vi "FuncImg-Export full data.vi"() -> (0 "error out":errorcluster, 11 "Exported file path":path)   [LabVIEW 2020]
uses:
  <userlib>/_MGI/File/MGI Windows Folder Enum.ctl
  Experiment header interface/Typedefs/Header parameters cluster-Zstack.ctl
  Typedefs/Frame Size.ctl
  Global variables/gl_Functional Imaging-Global variables.vi
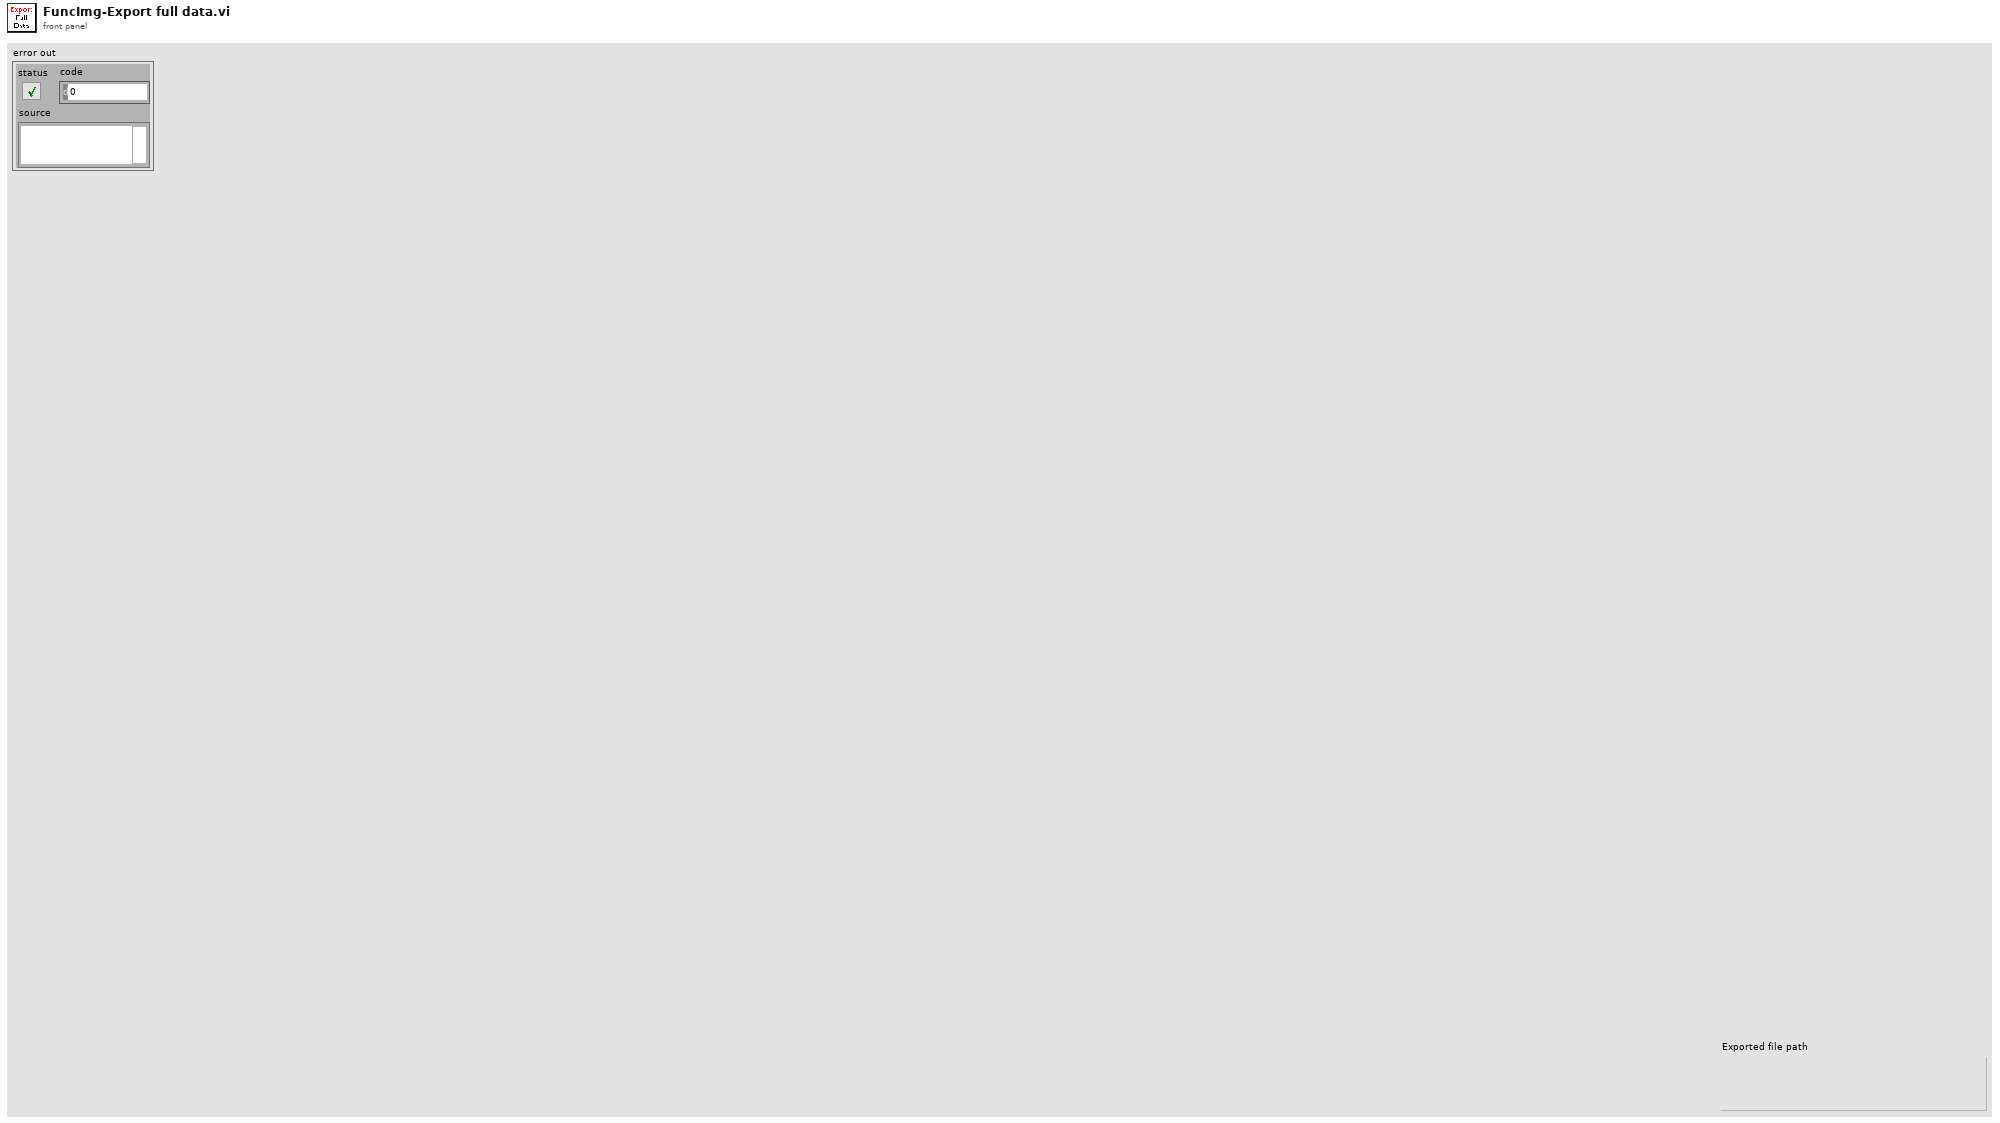
[diagram p1: front panel]
types:
  T1 = typedef "MGI Windows Folder Enum.ctl" = enum32{"Desktop", "Err<Internet>", "Programs", "Err<Controls>", "Err<Printers>", "Personal (MyDocuments)", "Favorites", "Startup", "Recent", "SendTo", "Err<RecycleBin>", "StartMenu", "Err<MyDocuments>", "MyMusic", "MyVideo", "Err<0x000F>", "DesktopDirectory", "Err<Drives>", "Err<Network>", "NetHood", "Fonts", "Templates", "CommonStartMenu", "CommonPrograms", "CommonStartup", "CommonDesktopDirectory", "AppData", "PrintHood", "LocalAppData", "Err<AltStartup>", "Err<CommonAltStartup>", "CommonFavorites", "InternetCache", "Cookies", "History", "CommonAppData", "Windows", "System", "ProgramFiles", "MyPictures", "Profile", "System32", "Err<0x002A>", "ProgramFilesCommon", "Err<0x002C>", "CommonTemplates", "CommonDocuments", "CommonAdminTools", "AdminTools"}
  T2 = enum16{"open", "open or create", "create or replace", "create", "open (read-only)"}
  T3 = typedef "Header parameters cluster-Zstack.ctl" = cluster{"Number of POI":u16, "Number of Miniscans":u16, "Number of Trials":u16, "Number of Cycles ":u16, "# Averaged Frames":u16, "Laser power (%)":u8, "Pockels":dbl, "Acquisition Length (sec)":dbl, "Fill time (us)":dbl, "DwellTime (us)":dbl, "Miniscan Dwell time per pixel (us)":dbl, "PMT 1":dbl, "PMT 2":dbl, "Back Apperture":dbl, "Zoom":dbl, "Number of Pixels in Miniscan":u16, "Frame Size":T4, "Field of View":dbl, "X centre":dbl, "Y centre":dbl, "AOL Z":dbl}
  T4 = typedef "Frame Size.ctl" = u16
  T5 = cluster{"Channel A?":bool, "MovCor enabled":bool, "Cycle time-stamps (us)":dbl[], "Cycle length (us)":dbl, "[Pixels in ROI]":i32[], "Z-Stack Header data":T3, "[ROI Time (us)]":dbl[], "Path out":path, "Version index":i32}
  T6 = typedef "Functional Imging UI Refs.ctl" = cluster{"Menu ref":refnum<k9>, "Image control":refnum<vi>, "VI ref":refnum<vi>, "XGrapher":refnum<vi>, "Smoothing":refnum<vi>, "POI Averaging":refnum<vi>, "Normalize":refnum<vi>, "POI data points in each trial":refnum<vi>, "Channel":refnum<vi>, "Experiment data folder path":refnum<vi>, "[ROI vis]":refnum<vi>, "[Groups] visbl":T7, "Group Name":refnum<vi>, "POI index":refnum<vi>, "Trial No.":refnum<vi>, "Intensity Zoom":refnum<vi>, "Trial Cursor Enabled":refnum<vi>, "Number of Trials (ind 1)":refnum<vi>, "Number of Trials (ind 2)":refnum<vi>, "MiniScans Available":refnum<vi>, "POI Available":refnum<vi>, "Defer graph updates":refnum<vi>, "Waveform selector":refnum<vi>, "#of selected POI":refnum<vi>, "#of selected MiniScans":refnum<vi>, "#of selected groups":refnum<vi>, "Max Z-Projection":refnum<vi>, "Z-Plane Selector":refnum<vi>, "Index of miniscan point to visualise":refnum<vi>, "ROI vis. mode":refnum<vi>, "Total # of points":refnum<vi>, "Index of group clicked on":refnum<vi>, "Pane 1":refnum<vi>, "Pane 2":refnum<vi>, "Pane 3":refnum<vi>, "Pane 4":refnum<vi>, "Pane 5":refnum<vi>, "Pane 6":refnum<vi>, "Deselect all ROI":refnum<vi>, "Deselect all groups":refnum<vi>}
  T7 = typedef "Groups array referecne.ctl" = refnum<vi>
  T8 = typedef "ROI selector array-ROI vis.ctl" = T9[]
  T9 = typedef "Interface-ROI selection cluster.ctl" = cluster{"ROI number":i32, "ROI ID":T10, "Visibility":bool}
  T10 = typedef "ROI ID Enum.ctl" = enum16{"Point", "MiniScan", "Comp. MiniScan", "Rectangle", "Comp. volume", "Arb. plane point", "None"}
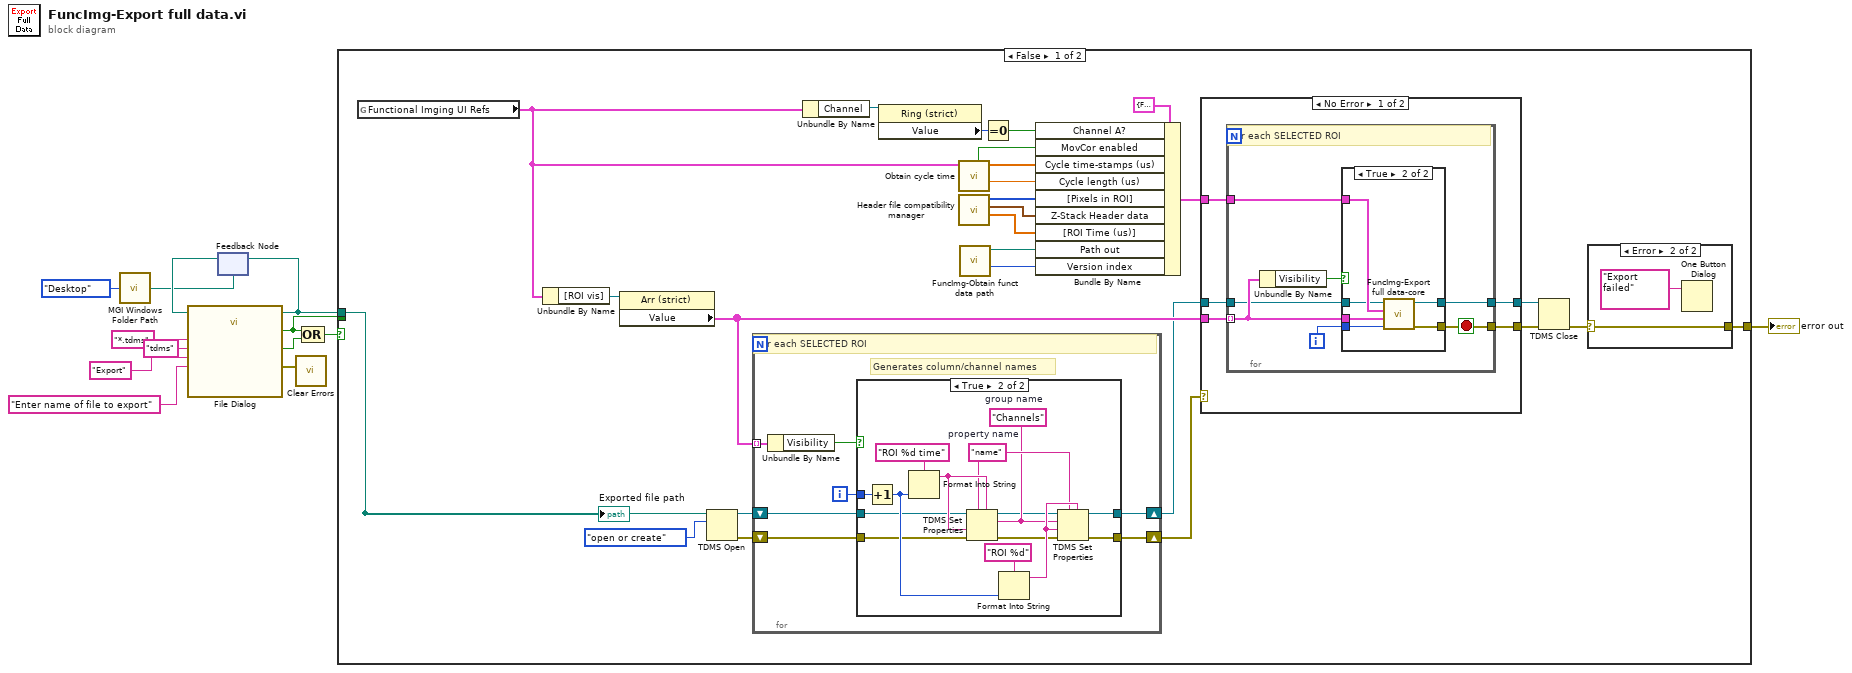
[diagram p0: block diagram]
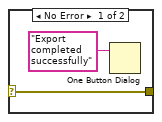
[diagram p2: hidden frame]
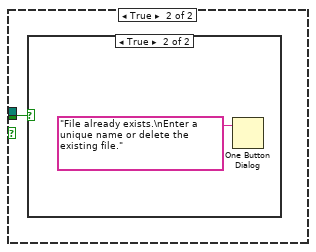
[diagram p6: hidden frame]
diagram:
  n1 = call <userlib>:"MGI Windows Folder Path.vi"("Windows Folder"=MGI_Windows_Folder_Enum."Desktop") -> ("Path"=w10:path)
  n2 = feedback #1(w10) -> (w12:path)
  n3 = call "File Dialog"("start path"=w12, "prompt"="Enter name of file to export", "button label"="Export", "pattern (all files)"="*.tdms" ("pattern label"), "pattern label"="tdms") -> ("selected path"=w1:path, "exists"=w2:bool, "cancelled"=w7:bool, "error out"=w8:errorcluster)  [unwired: 7 in]
  n4 = feedback-in #1(w1) -> ()
  n5 = call <vilib>:"Clear Errors.vi"("error in (no error)"=w8) -> ()  [unwired: 5 in, 2 out]
  n6 = Compound Arithmetic op=OR(w2, w7) -> (w6:bool)
  n7 = case shown="False" w6 {
    tunnel: [w14 _] -> w13
    tunnel: w2 -> [_ w88]
    tunnel: w1 -> [w16 _]
    frame False {
      n8 = global read "gl_Functional Imaging-Global variables.vi" "Functional Imging UI Refs"() -> (w29:T6)
      n9 = Unbundle By Name(w29) -> ("[ROI vis]"=w28:refnum<vi>)
      n10 = property on="Property Node" class="Arr (strict)"(reference=w28) -> ("Value"=w23:T8)  [unwired: 1 in, 2 out]
      n11 = TDMS Open(10:T2."open or create" ("operation (0:open)"), 11:w16) -> (0:w19:errorcluster, 3:w20:refnum<k34>)  [unwired: 5 in]
      n12 = for {
        tunnel: w23 -> [w71] mode=indexing
        shift-right: [w67] -> w18
        shift-left: w19 -> [w66]
        shift-right: [w65] -> w17
        shift-left: w20 -> [w68]
        i -> [w69]
        # "Generates column/channel names"
        # "For each SELECTED ROI"
        n13 = Unbundle By Name(w71) -> ("Visibility"=w70:bool)
        n14 = case shown="True" w70 {
          tunnel: w69 -> [_ w87]
          tunnel: w66 -> [w72 w78]
          tunnel: w68 -> [w73 w79]
          tunnel: [w73 w75] -> w65
          tunnel: [w72 w74] -> w67
          frame False {
          }
          frame True {
            w80 = "Channels"  # group name
            w81 = "name"  # property name
            n15 = Increment(x=w87) -> (x+1=w83:i32)
            n16 = Format Into String(format string="ROI %d time", w83) -> (resulting string=w82:string)  [unwired: 2 in, 1 out]
            n17 = TDMS Set Properties(5:w82, 7:w81, 8:w78, 9:w82, 10:w80, 11:w79) -> (0:w76:errorcluster, 3:w77:refnum<k34>)  [unwired: 2 out]
            n18 = Format Into String(format string="ROI %d", w83) -> (resulting string=w85:string)  [unwired: 2 in, 1 out]
            n19 = TDMS Set Properties(5:w85, 7:w81, 8:w76, 9:w85, 10:w80, 11:w77) -> (0:w74:errorcluster, 3:w75:refnum<k34>)  [unwired: 2 out]
          }
        }
      }
      n20 = Unbundle By Name(w29) -> ("Channel"=w27:refnum<vi>)
      n21 = property on="Property Node" class="Ring (strict)"(reference=w27) -> ("Value"=w38:u16)  [unwired: 1 in, 2 out]
      n22 = call "Obtain cycle time.vi"("Functional Imging UI Refs"=w29) -> ("Funct Acq cycle length (us)"=w32:dbl, "Single funct.acq cycle time-stamps (us) [MovCor only]"=w31:dbl[], "MovCor enabled (value from header file)"=w30:bool)  [unwired: 6 in, 2 out]
      n23 = call "Header file compatibility manager.vi"() -> ("[ROI Time (us)]"=w35:dbl[], "Z-Stack Header data"=w34:T3, "[Pixels in ROI]"=w26:i32[])  [unwired: 8 in, 1 out]
      n24 = call "FuncImg-Obtain funct data path.vi"() -> ("Version index (-1 = latest version)"=w37:i32, "Functional data folder path"=w36:path)  [unwired: 7 in, 3 out]
      n25 = Equal To 0?(x=w38) -> (x = 0?=w39:bool)
      n26 = Bundle By Name(cluster=T5 {"Channel A?"=FALSE, "MovCor enabled"=FALSE, "Cycle time-stamps (us)"=[], "Cycle length (us)"=0.0, "[Pixels in ROI]"=[], "Z-Stack Header data"={"Number of POI"=0, "Number of Miniscans"=0, "Number of Trials"=0, "Number of Cycles "=0, "# Averaged Frames"=0, "Laser power (%)"=0, "Pockels"=0.0, "Acquisition Length (sec)"=0.0, "Fill time (us)"=0.0, "DwellTime (us)"=0.0, "Miniscan Dwell time per pixel (us)"=0.0, "PMT 1"=0.0, "PMT 2"=0.0, "Back Apperture"=0.0, "Zoom"=0.0, "Number of Pixels in Miniscan"=0, "Frame Size"=200, "Field of View"=0.0, "X centre"=0.0, "Y centre"=0.0, "AOL Z"=0.0}, "[ROI Time (us)]"=[], "Path out"=path "", "Version index"=0} ("Cluster"), "Channel A?"=w39, "MovCor enabled"=w30, "Cycle time-stamps (us)"=w31, "Cycle length (us)"=w32, "[Pixels in ROI]"=w26, "Z-Stack Header data"=w34, "[ROI Time (us)]"=w35, "Path out"=w36, "Version index"=w37) -> (w25:T5)
      n27 = case shown="No Error" w18 {
        selector: w18 -> [_ w64]
        tunnel: [w48 w64] -> w21
        tunnel: w25 -> [w47 _]
        tunnel: w23 -> [w46 _]
        tunnel: w17 -> [w45 w63]
        tunnel: [w44 w63] -> w22
        frame No Error {
          n28 = for {
            tunnel: w46 -> [w53] mode=indexing
            tunnel: w47 -> [w55]
            tunnel: [w54] -> w48
            tunnel: w45 -> [w51]
            tunnel: [w49] -> w44
            i -> [w50]
            stop <- w54 stop-if-true
            # "For each SELECTED ROI"
            n29 = Unbundle By Name(w53) -> ("Visibility"=w52:bool)
            n30 = case shown="True" w52 {
              tunnel: w53 -> [_ w60]
              tunnel: w55 -> [_ w62]
              tunnel: [_ w61] -> w54
              tunnel: w51 -> [w56 w59]
              tunnel: w50 -> [_ w58]
              tunnel: [w56 w57] -> w49
              frame False {
              }
              frame True {
                n31 = call "FuncImg-Export full data-core.vi"("FOR loop index"=w58, "System Cluster"=w60, "Input cluster"=w62, "Exported tdms file"=w59) -> ("error out"=w61:errorcluster, "Exported tdms file"=w57:refnum<k34>)  [unwired: 6 in]
              }
            }
          }
        }
        frame Error {
        }
      }
      n32 = TDMS Close(8:w21, 11:w22) -> (0:w15:errorcluster)  [unwired: 1 out]
      n33 = case shown="Error" w15 {
        selector: w15 -> [w41 w43]
        tunnel: [w41 w43] -> w14
        frame No Error {
          n34 = One Button Dialog(message="Export completed successfully") -> ()  [unwired: 1 in, 1 out]
        }
        frame Error {
          n35 = One Button Dialog(message="Export failed") -> ()  [unwired: 1 in, 1 out]
        }
      }
      "Exported file path" <- w16
    }
    frame True {
      n36 = case shown="True" w88 {
        frame False {
        }
        frame True {
          n37 = One Button Dialog(message="File already exists.\nEnter a unique name or delete the existing file.") -> ()  [unwired: 1 in, 1 out]
        }
      }
    }
  }
  "error out" <- w13
